vi "Edit Icon 2011.vi"(8 "error in (no error)":errorcluster, 10 "Color 256 in":T1) -> (0 "error out":errorcluster, 2 "Color 256 out":T1)   [LabVIEW 2011]
uses:
  <vilib>/picture/picture.llb/imagedata.ctl
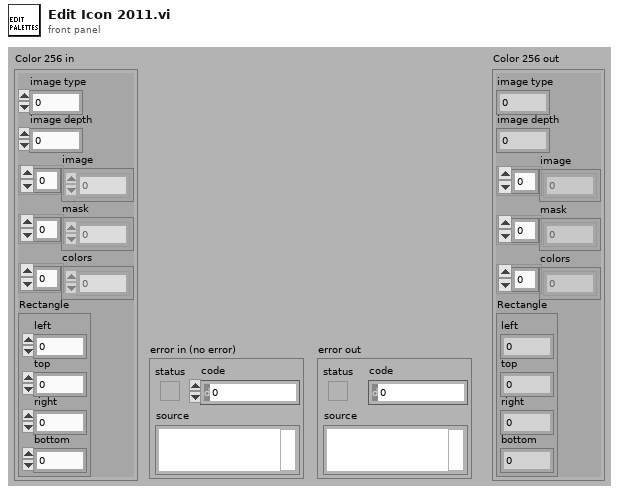
[diagram p1: front panel]
types:
  T1 = typedef "imagedata.ctl" = cluster{"image type":i32, "image depth":i32, "image":u8[], "mask":u8[], "colors":u32[], "Rectangle":cluster{"left":i16, "top":i16, "right":i16, "bottom":i16}}
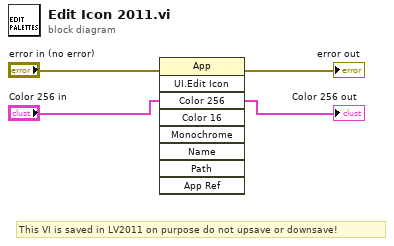
[diagram p0: block diagram]
diagram:
  # "This VI is saved in LV2011 on purpose do not upsave or downsave!"
  n1 = invoke class="App" method="UI.Edit Icon"(error in="error in (no error)", "Color 256"="Color 256 in") -> (error out=→"error out":errorcluster, "Color 256"=→"Color 256 out":T1)  [unwired: 7 in, 7 out]
